vi "Graphs.vi"() -> ()   [LabVIEW 2017]
uses:
  <vilib>/Platform/TimedLoop/XDataNode/timing_clust.ctl
  <vilib>/Platform/TimedLoop/XDataNode/nitl_modes.ctl
  <vilib>/Platform/TimedLoop/XDataNode/wakeup.ctl
  <vilib>/SWP/Math/Library/Polymorpic Source/DegressToRadiansDBL.vi
  <extravilib>/ChannelInstances/Tag-bool/Write With Abort.vi
  <extravilib>/ChannelInstances/Tag-bool/Read With Abort.vi
  <extravilib>/ChannelInstances/Tag-bool/Instantiate.vi
  <extravilib>/ChannelInstances/Event Messenger-u32/Instantiate.vi
  <extravilib>/ChannelInstances/Event Messenger-u32/))Channel.vi
  <extravilib>/ChannelInstances/Tag-bool/EndpointRead.vi
  <extravilib>/ChannelInstances/Event Messenger-dbl/Instantiate.vi
  <extravilib>/ChannelInstances/Event Messenger-dbl/))Channel.vi
  <extravilib>/ChannelInstances/Tag-bool/Endpoint.vi
  <vilib>/platform/TimedLoop/XDataNode/XDataNode.xnode
  <vilib>/Platform/TimedLoop/XDataNode/XDNodeRunTimeDep.lvlib
  <extravilib>/ChannelInstances/Event Messenger-dbl.lvlib
  <extravilib>/ChannelInstances/Event Messenger-u32.lvlib
  <extravilib>/ChannelInstances/Tag-bool.lvlib
  <vilib>/SWP/Math/Math.lvlib
panel:
  out "Waveform Chart 3":dbl(graph)
  out "Waveform Chart 2":dbl(graph)
  out "Waveform Chart":u32(graph)
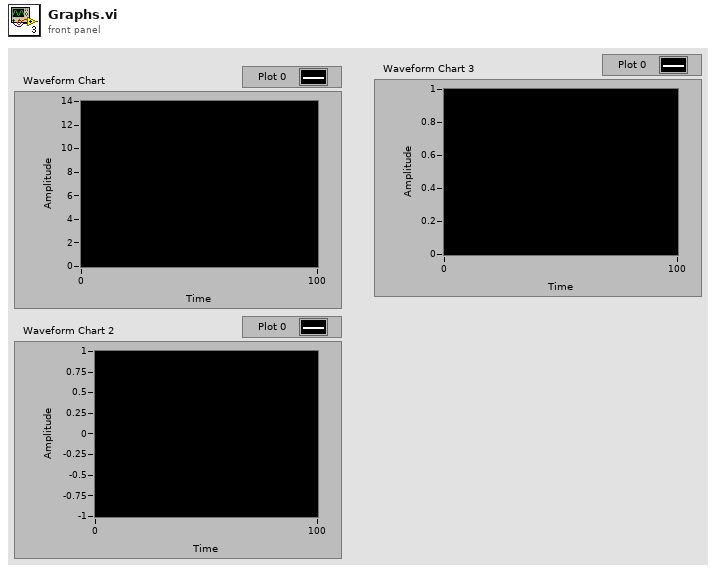
[diagram p1: front panel]
types:
  T1 = typedef "XDNodeRunTimeDep.lvlib/timing_clust.ctl" = cluster{"Expected End [f-1]":u64, "Actual End [f-1]":u64, "Finished Late? [f-1]":bool, "Expected End [i-1]":u64, "Actual End [i-1]":u64, "Finished Late? [i-1]":bool, "Expected Start [i]":u64, "Actual Start [i]":u64, "Expected Start [f]":u64, "Actual Start [f]":u64, "Source Name":string, "Structure Name":string, "Period":i64, "Deadline":i64, "Offset":i64, "Start":i64, "Priority":i32, "Timeout":i32, "Mode":T2, "Wakeup Reason":T3, "Error":errorcluster, "Source Type":string, "Secondary Source Type":string, "Global End Time":u64, "Global Start Time":u64, "Frame Duration":u64, "Iteration Duration":u64, "Assigned CPU":i32, "I/O Scan Engine Mode":u32}
  T2 = typedef "XDNodeRunTimeDep.lvlib/nitl_modes.ctl" = enum32{"No Change", "Process missed periods, maintain original phase", "Discard missed periods, maintain original phase", "Process missed periods, ignore original phase", "Discard missed periods, ignore original phase"}
  T3 = typedef "XDNodeRunTimeDep.lvlib/wakeup.ctl" = enum32{"Normal", "Aborted", "Asynchronous wakeup", "Timing source error", "Timed loop error", "Timeout"}
  T4 = typedef "Event Messenger-u32.lvlib/))Channel.ctl" = refnum<queue>
  T5 = typedef "Event Messenger-dbl.lvlib/))Channel.ctl" = refnum<queue>
  T6 = cluster{"event registration refnum":refnum<event-registration>, "event registration refnum":refnum<event-registration>, "event registration refnum":refnum<event-registration>}
  T7 = typedef "Tag-bool.lvlib/))Channel.ctl" = refnum<queue>
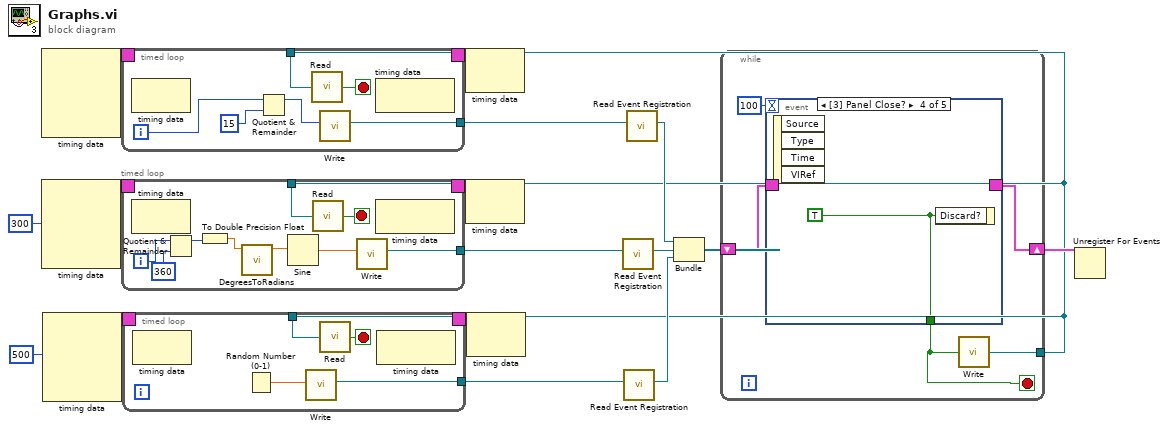
[diagram p0: block diagram]
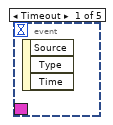
[diagram p2: hidden frame]
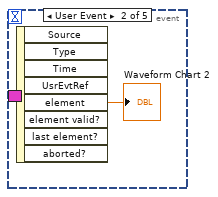
[diagram p3: hidden frame]
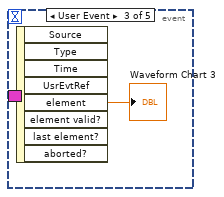
[diagram p4: hidden frame]
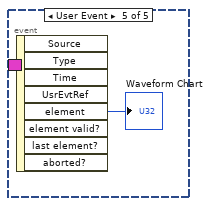
[diagram p5: hidden frame]
diagram:
  n1 = node-c288() -> (w17:T1)  [unwired: 4 in]
  n2 = node-c288(i64 300 ("Period")) -> (w15:T1)  [unwired: 3 in]
  n3 = node-c288(i64 500 ("Period")) -> (w12:T1)  [unwired: 3 in]
  n4 = timed-loop {
    timing: w17 -> [_]
    timing-out: [_] -> w16
    tunnel: [w21] -> w7
    tunnel: w1 -> [w19]
    i -> [w20]
    stop <- w18 stop-if-true
    n5 = node-c288() -> ()  [unwired: 1 in, 1 out]
    n6 = Quotient & Remainder(x=w20, y=u32 15) -> (x-y*floor(x/y)=w22:u32)  [unwired: 1 out]
    n7 = call <extravilib>:"Read.vi"("channel"=w19) -> ("element"=w18:bool)  [unwired: 1 in, 1 out]
    n8 = call <extravilib>:"Write.vi"("element"=w22) -> ("channel"=w21:T4)  [unwired: 9 in, 1 out]
    n9 = node-c288() -> ()  [unwired: 1 in, 1 out]
  }
  n10 = node-c288(w16) -> ()  [unwired: 1 out]
  n11 = call <extravilib>:"Read Event Registration.vi"("channel"=w7) -> ("event registration refnum"=w6:refnum<event-registration>)  [unwired: 10 in]
  n12 = timed-loop {
    timing: w15 -> [_]
    timing-out: [_] -> w14
    tunnel: [w32] -> w8
    tunnel: w1 -> [w28]
    i -> [w31]
    stop <- w29 stop-if-true
    n13 = node-c288() -> ()  [unwired: 1 in, 1 out]
    n14 = Quotient & Remainder(x=w31, y=u32 360) -> (x-y*floor(x/y)=w30:u32)  [unwired: 1 out]
    n15 = To Double Precision Float(number=w30) -> (double precision float=w27:dbl)
    n16 = call-poly <vilib>:"DegreesToRadians.vi"("Degrees"=w27) -> ("Radians"=w26:dbl)  [unwired: 9 in, 1 out]
    n17 = Sine(x=w26) -> (sin(x)=w33:dbl)
    n18 = call <extravilib>:"Read.vi"("channel"=w28) -> ("element"=w29:bool)  [unwired: 1 in, 1 out]
    n19 = call <extravilib>:"Write.vi"("element"=w33) -> ("channel"=w32:T5)  [unwired: 9 in, 1 out]
    n20 = node-c288() -> ()  [unwired: 1 in, 1 out]
  }
  n21 = node-c288(w14) -> ()  [unwired: 1 out]
  n22 = call <extravilib>:"Read Event Registration.vi"("channel"=w8) -> ("event registration refnum"=w5:refnum<event-registration>)  [unwired: 10 in]
  n23 = timed-loop {
    timing: w12 -> [_]
    timing-out: [_] -> w11
    tunnel: [w39] -> w9
    tunnel: w1 -> [w37]
    stop <- w38 stop-if-true
    n24 = node-c288() -> ()  [unwired: 1 in, 1 out]
    n25 = Random Number (0-1)() -> (number: 0 to 1=w40:dbl)
    n26 = call <extravilib>:"Write.vi"("element"=w40) -> ("channel"=w39:T5)  [unwired: 9 in, 1 out]
    n27 = call <extravilib>:"Read.vi"("channel"=w37) -> ("element"=w38:bool)  [unwired: 1 in, 1 out]
    n28 = node-c288() -> ()  [unwired: 1 in, 1 out]
  }
  n29 = node-c288(w11) -> ()  [unwired: 1 out]
  n30 = call <extravilib>:"Read Event Registration.vi"("channel"=w9) -> ("event registration refnum"=w4:refnum<event-registration>)  [unwired: 10 in]
  n31 = Bundle("event registration refnum"=w6, "event registration refnum"=w5, "event registration refnum"=w4) -> (w3:T6)  [unwired: 1 in]
  n32 = while {
    shift-right: [w46] -> w2
    shift-left: w3 -> [w47]
    tunnel: [w43] -> w1
    stop <- w45 stop-if-true
    n33 = event shown="[3] Panel Close?" {
      selector: w47 -> [_ _ _ _ _]
      dyn-events: [_ _ _ _ _] -> w46
      timeout: 100 -> [_ _ _ _ _]
      tunnel: [_ _ _ w50 _] -> w45
      event Timeout {
        n34 = event-data() -> ()  [unwired: 1 in, 3 out]
      }
      event User Event {
        n35 = event-data() -> ("element"=→"Waveform Chart 2":dbl)  [unwired: 1 in, 7 out]
      }
      event User Event {
        n36 = event-data() -> ("element"=→"Waveform Chart 3":dbl)  [unwired: 1 in, 7 out]
      }
      event Panel Close? {
        w50 = TRUE ("Discard?")
        n37 = event-data() -> ()  [unwired: 1 in, 4 out]
        n38 = event-data("Discard?"=w50) -> ()  [unwired: 1 in, 1 out]
      }
      event User Event {
        n39 = event-data() -> ("element"=→"Waveform Chart":u32)  [unwired: 1 in, 7 out]
      }
    }
    n40 = call <extravilib>:"Write.vi"("element"=w45) -> ("channel"=w43:T7)  [unwired: 1 out]
  }
  n41 = Unregister For Events(event registration refnum=w2) -> ()  [unwired: 1 in, 1 out]
